vi "Create From Variant.vi"(8 "error in (no error)":errorcluster, 10 "Variant":variant, 11 "JSON Numeric in":refnum<class "JSON Numeric.lvclass">) -> (0 "error out":errorcluster, 3 "JSON Numeric out":refnum<class "JSON Numeric.lvclass">)   [LabVIEW 2015, in "LVJSON.lvlib" / "JSON Numeric.lvclass"]
doc: "Creates a new JSON instance from the given Variant."
uses:
  JSON Numeric.lvclass
  JSON Numeric.lvclass/JSON Numeric.ctl
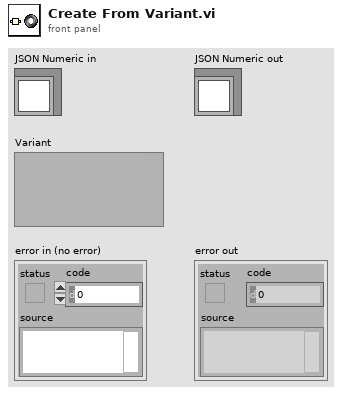
[diagram p1: front panel]
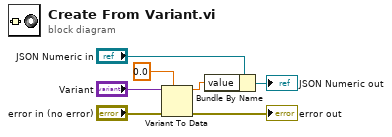
[diagram p0: block diagram]
diagram:
  n1 = Variant To Data(error in="error in (no error)", type=0.0, Variant="Variant") -> (data=w4:dbl, error out=→"error out":errorcluster)
  n2 = Bundle By Name(cluster="JSON Numeric in", "value"=w4) -> (→"JSON Numeric out":refnum<class "JSON Numeric.lvclass">)
